vi "Motor Controller One-shot data.vi"(10 "RS-485 addr.":u8=1 min=1, 11 "COM port":refnum<visa-resource-name>) -> (0 "Error out":errorcluster, 1 "Checksum ok":bool, 2 "Frame ok":bool, 3 "Data cluster":T1)   [LabVIEW 2020]
uses:
  ctls/CTRL_Data_Out.ctl
  ctls/CTRL_Cmd.ctl
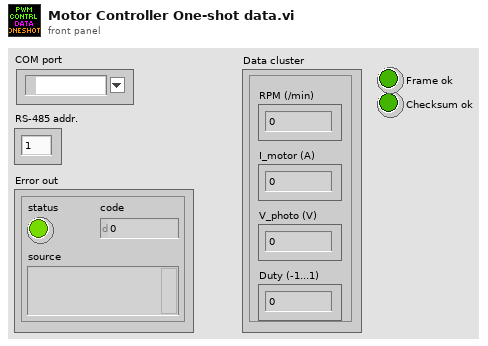
[diagram p1: front panel]
types:
  T1 = typedef "CTRL_Data_Out.ctl" = cluster{"RPM (/min)":sgl, "I_motor (A)":sgl, "V_photo (V)":sgl, "Duty (-1...1)":sgl}
  T2 = typedef "CTRL_Cmd.ctl" = string
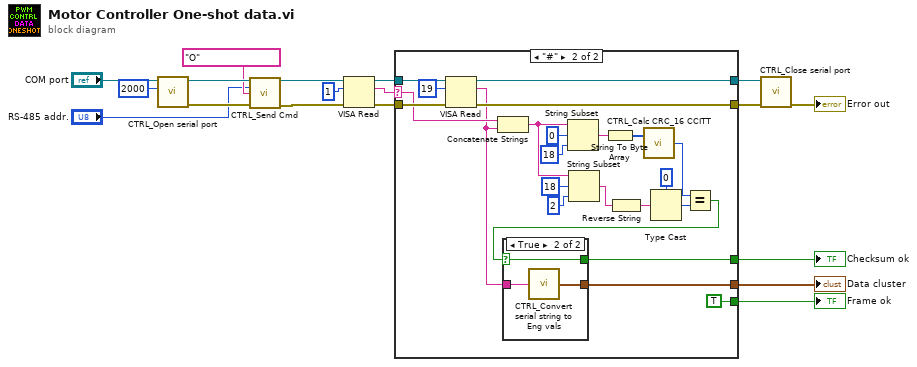
[diagram p0: block diagram]
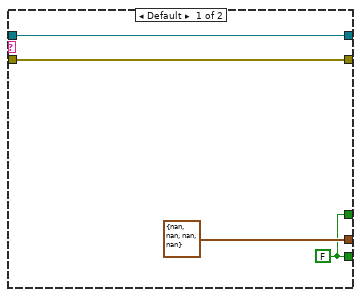
[diagram p2: hidden frame]
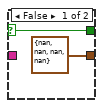
[diagram p3: hidden frame]
diagram:
  n1 = call "CTRL_Open serial port.vi"("timeout (ms)"=u32 2000, "VISA resource name"="COM port") -> ("Error out"=w6:errorcluster, "VISA resource name out"=w14:refnum<visa-resource-name>)  [unwired: 8 in]
  n2 = call "CTRL_Send Cmd.vi"("Port"=w14, "RS-485 addr."="RS-485 addr.", "Cmd"=T2 "O" ("Command"), "Error In"=w6) -> ("Port out"=w15:refnum<visa-resource-name>, "Error Out"=w16:errorcluster)  [unwired: 10 in]
  n3 = VISA Read(VISA resource name=w15, byte count=u32 1, error in (no error)=w16) -> (VISA resource name out=w9:refnum<visa-resource-name>, read buffer=w8:string, error out=w10:errorcluster)  [unwired: 1 out]
  n4 = case shown="\"#\"" w8 {
    selector: w8 -> [_ w40]
    tunnel: w10 -> [w22 w44]
    tunnel: w9 -> [w21 w45]
    tunnel: [w22 w42] -> w5
    tunnel: [w21 w41] -> w4
    tunnel: [T1 {"RPM (/min)"=nan, "I_motor (A)"=nan, "V_photo (V)"=nan, "Duty (-1...1)"=nan} ("Data") w25] -> w12
    tunnel: [w19 w24] -> w3
    tunnel: [w19 TRUE] -> w2
    frame Default {
      w19 = FALSE
    }
    frame "#" {
      n5 = VISA Read(VISA resource name=w45, byte count=u32 19, error in (no error)=w44) -> (VISA resource name out=w41:refnum<visa-resource-name>, read buffer=w39:string, error out=w42:errorcluster)  [unwired: 1 out]
      n6 = Concatenate Strings(w40, w39) -> (w27:string)
      n7 = String Subset(string=w27, offset (0)=0, length (rest)=18 ("length (rest)")) -> (substring=w26:string)
      n8 = String Subset(string=w27, offset (0)=18, length (rest)=2 ("length (rest)")) -> (substring=w35:string)
      n9 = String To Byte Array(string=w26) -> (unsigned byte array=w38:u8[])
      n10 = Reverse String(1:w35) -> (0:w33:string)
      n11 = call "CTRL_Calc CRC_16 CCITT.vi"("Data bytes"=w38) -> ("CRC_16-CCITT"=w32:u16)  [unwired: 1 in]
      n12 = Type Cast(type=u16 0 ("length (rest)"), x=w33) -> (*(type *) &x=w31:u16)
      n13 = Equal?(x=w32, y=w31) -> (x = y?=w30:bool)
      n14 = case shown="True" w30 {
        selector: w30 -> [w46 w48]
        tunnel: w39 -> [_ w50]
        tunnel: [T1 {"RPM (/min)"=nan, "I_motor (A)"=nan, "V_photo (V)"=nan, "Duty (-1...1)"=nan} ("Data") w49] -> w25
        tunnel: [w46 w48] -> w24
        frame False {
        }
        frame True {
          n15 = call "CTRL_Convert serial string to Eng vals.vi"("Serial buffer string (excluding FrameChar)"=w50) -> ("Data"=w49:T1)
        }
      }
    }
  }
  "Data cluster" <- w12
  "Checksum ok" <- w3
  "Frame ok" <- w2
  n16 = call "CTRL_Close serial port.vi"("Error in"=w5, "VISA resource name"=w4) -> ("Error out"=→"Error out":errorcluster)  [unwired: 9 in]
